vi "Shutdown.vi"(8 "error in":errorcluster, 11 "MLTFNC in":refnum<class "MLTFNC.lvclass">) -> (0 "error out":errorcluster, 3 "MLTFNC out":refnum<class "MLTFNC.lvclass">)   [LabVIEW 2019, in "MLTFNC.lvlib" / "MLTFNC.lvclass"]
uses:
  Library/MLTFNC.lvclass
  builds/Instruments/Instruments.lvlibp/Library/Instruments.lvclass
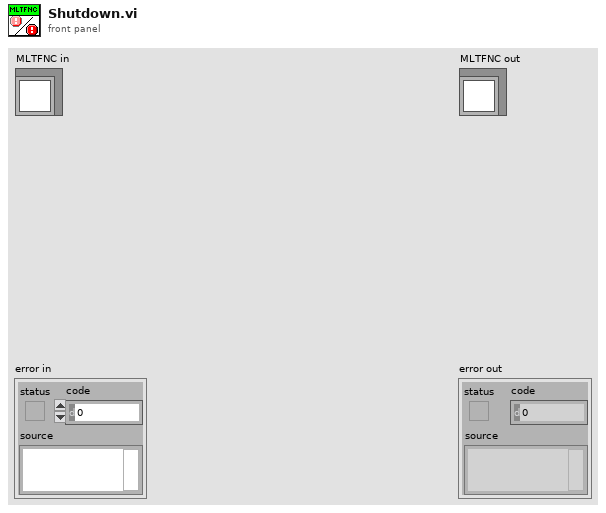
[diagram p1: front panel]
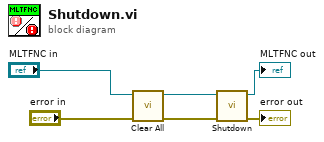
[diagram p0: block diagram]
diagram:
  n1 = call-dynamic "Clear All.vi"("error in"="error in", "MLTFNC in"="MLTFNC in") -> ("error out"=w3:errorcluster, "MLTFNC out"=w2:refnum<class "MLTFNC.lvclass">)  [unwired: 8 in]
  n2 = call-parent "Shutdown.vi"("error in"=w3, "Instruments in"=w2) -> ("error out"=→"error out":errorcluster, "Instruments out"=→"MLTFNC out":refnum<class "MLTFNC.lvclass">)  [unwired: 8 in]
